vi "New Pulse Acquired.vi"(8 "error in (no error)":errorcluster, 9 "Open plot":bool, 10 "Result in":refnum<class "Acquired Result.lvclass">, 11 "LabActor in":refnum<class "LabActor.lvclass">) -> (0 "error out":errorcluster, 3 "LabActor out":refnum<class "LabActor.lvclass">)   [LabVIEW 2021, in "LabActor.lvclass"]
uses:
  LabActor.lvclass
  NHMFL_Core/Libraries/Instruments/Results/Acquired Result/Acquired Result.lvclass
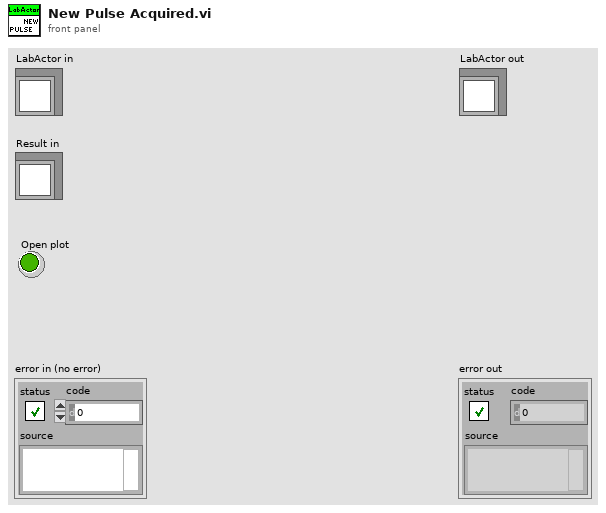
[diagram p1: front panel]
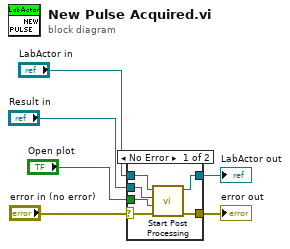
[diagram p0: block diagram]
diagram:
  n1 = case shown="No Error" "error in (no error)" {
    selector: "error in (no error)" -> [w7 w14]
    tunnel: [w10 w14] -> w5
    tunnel: [w11 w13] -> w3
    tunnel: "LabActor in" -> [w12 w13]
    tunnel: "Result in" -> [w8 _]
    tunnel: "Open plot" -> [w9 _]
    frame No Error {
      n2 = call-dynamic "Start Post Processing.vi"("error in (no error)"=w7, "Open plot"=w9, "Result in"=w8, "Application Controller in"=w12) -> ("error out"=w10:errorcluster, "Application Controller out"=w11:refnum<class "LabActor.lvclass">)  [unwired: 5 in, 1 out]
    }
    frame Error {
    }
  }
  "error out" <- w5
  "LabActor out" <- w3
